vi "Extract ROI Info.vi"(11 "AVI File Path":path) -> (1 "No of Patches in each Volume":i32[](array[numeric]), 2 "No of  ROIs":dbl, 3 "ROI ID":dbl, 5 "ROI setup":T1[](array[typedef]) {"Apparent Frame Size" format="%#_6f"; "Original FOV (um)" format="%#_6f"; "Pixels per miniscan" format="%#_6f"; "Dwell Time per pixel" format="%#_6f"; "Resolution" format="%#_6f"; "ROI group ID" format="%#_6f"; "Laser Power (%)" format="%#_6f"; "Zoom" format="%#_6f"; "Frame Size" format="%#_6f"; "Number of lines" format="%#_6f"; "Composite ID" format="%#_6f"; "Angle (deg)" format="%#_6f"; "ROI Time (ns)" format="%#_6f"; "ROI ID" format="%#_6f"; "Pixels in ROI" format="%#_6f"; "ROI index" format="%#_6f"; "Z stop" format="%#_6f"; "Y stop" format="%#_6f"; "X stop" format="%#_6f"; "Z start" format="%#_6f"; "X start" format="%#_6f"; "Y start" format="%#_6f"})   [LabVIEW 2020]
uses:
  Functional Imaging Viewer/Typedefs/ROI parameters data type.ctl
  <userlib>/_OpenG.lib/array/array.llb/Filter 1D Array (I32)__ogtk.vi
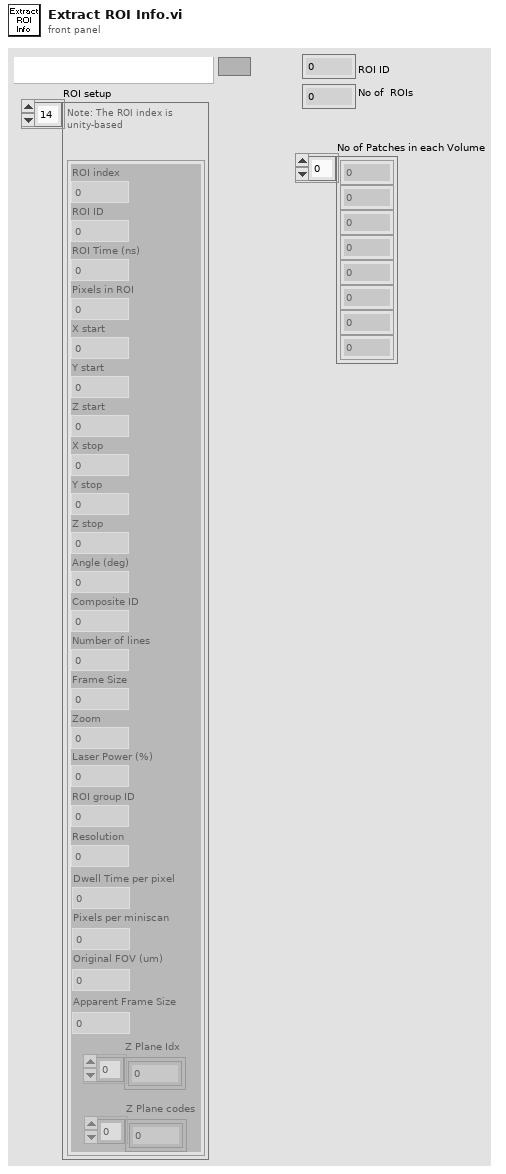
[diagram p1: front panel]
types:
  T1 = typedef "ROI parameters data type.ctl" = cluster{"ROI index":dbl, "ROI ID":dbl, "ROI Time (ns)":dbl, "Pixels in ROI":dbl, "X start":dbl, "Y start":dbl, "Z start":dbl, "X stop":dbl, "Y stop":dbl, "Z stop":dbl, "Angle (deg)":dbl, "Composite ID":dbl, "Number of lines":dbl, "Frame Size":dbl, "Zoom":dbl, "Laser Power (%)":dbl, "ROI group ID":dbl, "Resolution":dbl, "Dwell Time per pixel":dbl, "Pixels per miniscan":dbl, "Original FOV (um)":dbl, "Apparent Frame Size":dbl, "Z Plane Idx":i32[], "Z Plane codes":i32[]}
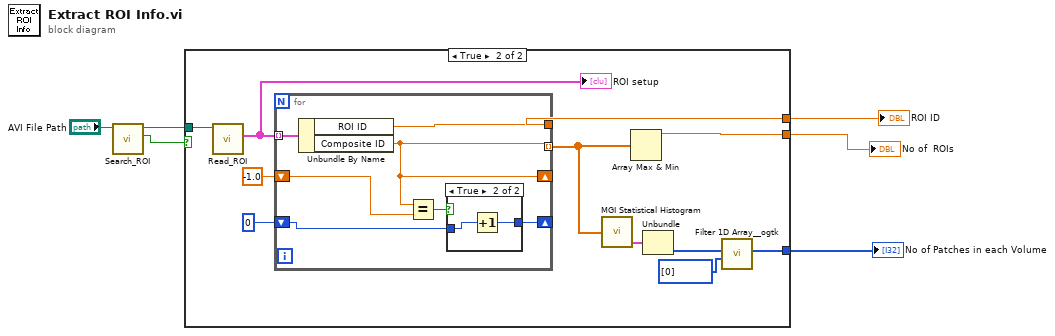
[diagram p0: block diagram]
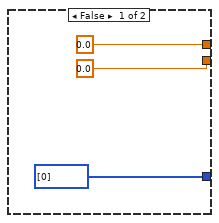
[diagram p2: hidden frame]
diagram:
  n1 = call "Search_ROI.vi"("AVI File Path"="AVI File Path") -> ("ROI File Exists"=w4:bool, "ROI Path"=w6:path)  [unwired: 9 in]
  n2 = case shown="True" w4 {
    tunnel: w6 -> [_ w20]
    tunnel: [0.0 w18] -> w2
    tunnel: [0.0 ("ROI ID") w17] -> w3
    tunnel: [i32[] [0] w11] -> w1
    frame False {
    }
    frame True {
      n3 = call "Read_ROI.vi"("Experiment folder path"=w20) -> ("ROI setup"=w19:T1[])  [unwired: 9 in, 1 out]
      "ROI setup" <- w19
      n4 = for {
        tunnel: w19 -> [w27] mode=indexing
        tunnel: [w26] -> w17
        tunnel: [w23] -> w14 mode=indexing
        shift-right: [w21] -> _
        shift-left: 0 -> [w22]
        shift-right: [w23] -> _
        shift-left: -1.0 ("Composite ID") -> [w24]
        n5 = Unbundle By Name(w27) -> ("ROI ID"=w26:dbl, "Composite ID"=w23:dbl)
        n6 = Equal?(x=w23, y=w24) -> (x = y?=w25:bool)
        n7 = case shown="True" w25 {
          tunnel: w22 -> [_ w29]
          tunnel: [_ w28] -> w21
          frame False {
          }
          frame True {
            n8 = Increment(x=w29) -> (x+1=w28:i32)
          }
        }
      }
      n9 = call <userlib>:"MGI Statistical Histogram.vi"("X[]"=w14) -> ("Histogram"=w13:cluster{dbl, "standard deviation":dbl, i32[]})  [unwired: 2 out]
      n10 = Array Max & Min(array=w14) -> (max value=w18:dbl)  [unwired: 3 out]
      n11 = Unbundle(w13) -> (w10:i32[])  [unwired: 2 out]
      n12 = call-poly <userlib>:"Filter 1D Array__ogtk.vi"("items to filter"=i32[] [0], "array"=w10) -> ("filtered array"=w11:i32[])  [unwired: 4 in, 1 out]
    }
  }
  "No of  ROIs" <- w2
  "ROI ID" <- w3
  "No of Patches in each Volume" <- w1
